vi "tcsWEP_acceptCommand_standby.vi"(8 "error in (no error)":errorcluster, 11 "command_standby_Ctl":T1) -> (0 "error out":errorcluster, 2 "function return":i32, 3 "command_standby_Ctl out":T1)   [LabVIEW 2016, in "SALLV_tcsWEP.lvlib"]
doc: "int tcsWEP_shm_acceptCommand_standbyLV(tcsWEP_command_standbyLV *command_standby_Ctl );"
uses:
  SALLV_tcsWEP.lvlib
  DataTypes/command_standby.ctl
  SALLV_tcsWEP.so
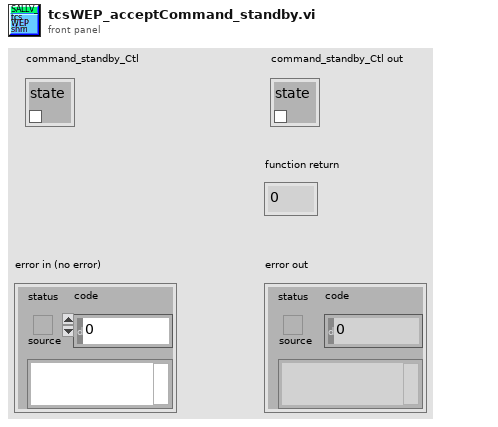
[diagram p1: front panel]
types:
  T1 = typedef "SALLV_tcsWEP.lvlib/command_standby.ctl" = cluster{"state":bool}
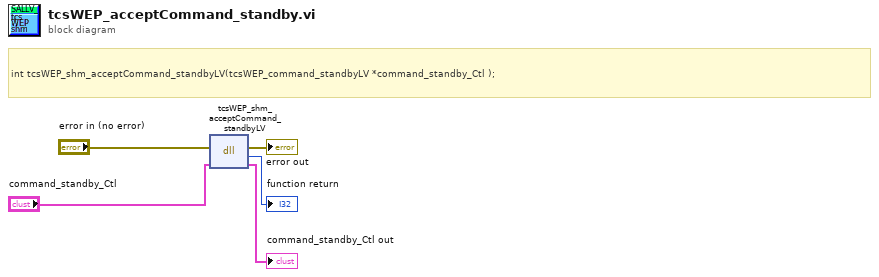
[diagram p0: block diagram]
diagram:
  # "int tcsWEP_shm_acceptCommand_standbyLV(tcsWEP_command_standbyLV *command_standby_Ctl );"
  n1 = dll-call lib="home/ttsai/Documents/salAPI/SALLV_tcsWEP.*" fn="tcsWEP_shm_acceptCommand_standbyLV"(error in="error in (no error)", "command_standby_Ctl"="command_standby_Ctl") -> (error out=→"error out":errorcluster, →"function return":i32, "command_standby_Ctl"=→"command_standby_Ctl out":T1)  [unwired: 2 in, 1 out]
